vi "Tx Inline Start.vi"(8 "error in (no error)":errorcluster, 10 "Dispatcher Interface in":refnum<class "Dispatcher Interface.lvclass">, 11 "Plugin in":refnum<class "Plugin.lvclass">) -> (0 "error out":errorcluster, 2 "Dispatcher Interface out":refnum<class "Dispatcher Interface.lvclass">, 3 "Plugin out":refnum<class "Plugin.lvclass">)   [LabVIEW 2019, in "DSF Core.lvlib" / "Plugin.lvclass"]
uses:
  Plugin.lvclass
  Interface/Dispatcher/Dispatcher Interface.lvclass
  Plugin.lvclass/Plugin.ctl
  Interface/Dispatcher/Command.ctl
  Transfer Group/Transfer Group.lvclass/Transfer Group.ctl
  Transfer Group/Transfer Group.lvclass
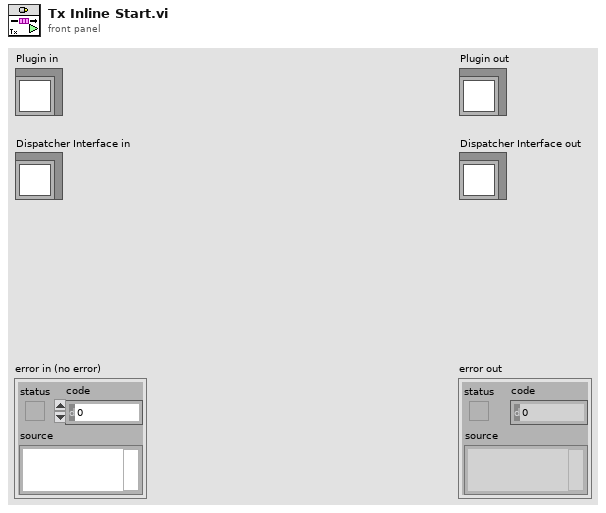
[diagram p1: front panel]
types:
  T1 = typedef "DSF Core.lvlib/Dispatcher Interface.lvclass/Command.ctl" = enum8{"Idle", "Start", "Rx", "Tx", "Set Inline Buffer", "Shutdown", "Error"}
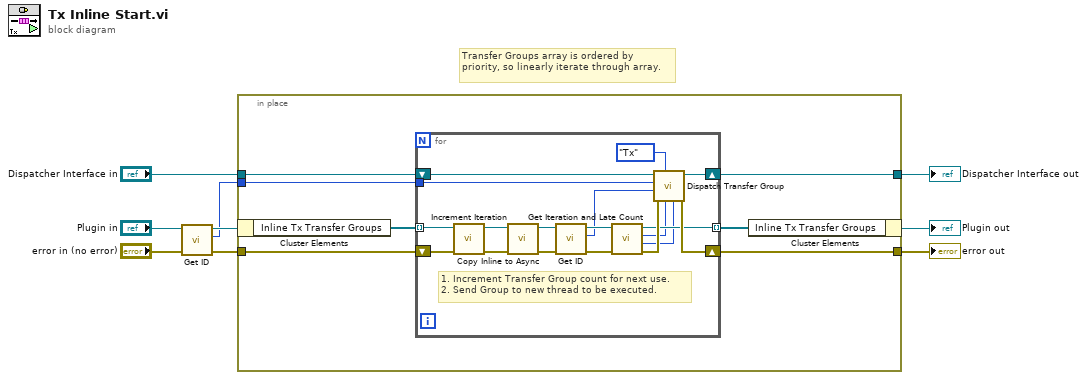
[diagram p0: block diagram]
diagram:
  # "Transfer Groups array is ordered by priority, so linearly iterate through array."
  n1 = call "Get ID.vi"("Plugin in"="Plugin in") -> ("id"=w2:i32, "Plugin out"=w3:refnum<class "Plugin.lvclass">)  [unwired: 9 in]
  n2 = in-place {
    in-place-border: "error in (no error)" -> [w15]
    in-place-border: [w14] -> w7
    in-place-border: "Dispatcher Interface in" -> [w11]
    in-place-border: w2 -> [w10]
    in-place-border: [w9] -> w1
    n3 = in-place-cluster #1(w3) -> ("Inline Tx Transfer Groups"=w13:refnum<class "Transfer Group.lvclass">[])
    n4 = for {
      tunnel: w13 -> [w32] mode=indexing
      shift-right: [w24] -> w14
      shift-left: w15 -> [w31]
      tunnel: [w23] -> w12 mode=indexing
      shift-right: [w27] -> w9
      shift-left: w11 -> [w26]
      tunnel: w10 -> [w18]
      # "1. Increment Transfer Group count for next use.\n2. Send Group to new thread to be executed."
      n5 = call "Increment Iteration.vi"("error in (no error)"=w31, "Transfer Group in"=w32) -> ("error out"=w29:errorcluster, "Transfer Group out"=w30:refnum<class "Transfer Group.lvclass">)  [unwired: 8 in]
      n6 = call "Copy Inline to Async.vi"("error in (no error)"=w29, "Transfer Group in"=w30) -> ("error out"=w28:errorcluster, "Transfer Group out"=w21:refnum<class "Transfer Group.lvclass">)  [unwired: 8 in]
      n7 = call "Get ID.vi"("Transfer Group in"=w21) -> ("id"=w19:i32, "Transfer Group out"=w20:refnum<class "Transfer Group.lvclass">)  [unwired: 9 in]
      n8 = call "Get Iteration and Late Count.vi"("error in (no error)"=w28, "Transfer Group in"=w20) -> ("error out"=w25:errorcluster, "late count"=w16:i32, "iteration"=w22:u64, "Transfer Group out"=w23:refnum<class "Transfer Group.lvclass">)  [unwired: 6 in]
      n9 = call "Dispatch Transfer Group.vi"("Late Count"=w16, "Iteration"=w22, "command"=Command."Tx", "error in (no error)"=w25, "Transfer Group ID"=w19, "Plugin ID"=w18, "Dispatcher Interface in"=w26) -> ("error out"=w24:errorcluster, "Dispatcher Interface out"=w27:refnum<class "Dispatcher Interface.lvclass">)  [unwired: 3 in]
    }
    n10 = in-place-cluster #1("Inline Tx Transfer Groups"=w12) -> (→"Plugin out":refnum<class "Plugin.lvclass">)
  }
  "error out" <- w7
  "Dispatcher Interface out" <- w1
